vi "Test.vi"   [LabVIEW 2024]
uses:
  DAQmx Actor/Analog Reader/Analog Reader.lvclass
  <vilib>/DAQmx/create/channels.llb/DAQmx Create Channel (AI-Voltage-Basic).vi
  <vilib>/DAQmx/configure/timing.llb/DAQmx Timing (Sample Clock).vi
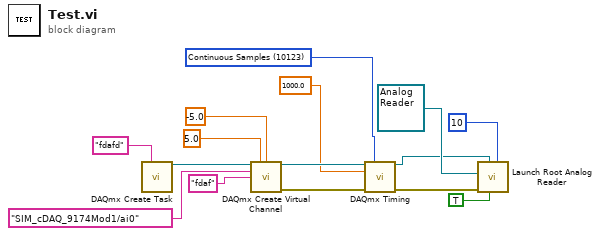
[diagram p0: block diagram]
diagram:
  w13 = 10123 items=["Finite Samples"=10178, "Continuous Samples"=10123, "Hardware Timed Single Point"=12522] ("sample mode")
  n1 = call <vilib>:"DAQmx Create Task.vi"("new task name"="fdafd") -> ("task out"=w2:refnum<k21>)  [unwired: 13 in, 1 out]
  n2 = call-poly <vilib>:"DAQmx Create Virtual Channel.vi"("task in"=w2, "maximum value"=5.0, "minimum value"=-5.0, "physical channels"=tag "SIM_cDAQ_9174Mod1/ai0", "name to assign"="fdaf") -> ("task out"=w15:refnum<k21>, "error out"=w8:errorcluster)  [unwired: 9 in]
  n3 = call-poly <vilib>:"DAQmx Timing.vi"("task/channels in"=w15, "sample mode"=w13, "rate"=1000.0, "error in"=w8) -> ("task out"=w4:refnum<k21>, "error out"=w7:errorcluster)  [unwired: 10 in]
  n4 = call "Launch Root Analog Reader.vi"("Loop Period in ms (10)"=u32 10, "Open Actor Core front panel? (F)"=TRUE, "DAQmx Task"=w4, "error in (no error)"=w7, "Analog Reader"=refnum<class "Analog Reader.lvclass"> refnum) -> ()  [unwired: 5 in, 2 out]
